vi "Configure_Voltage.vi"(6 "Measurement Type":T2(ring), 8 "error in (no error)":errorcluster, 9 "Resolution in Digits":T1(ring), 10 "Range":dbl=1.2, 11 "NI-DMM in":refnum<class "niDMM.lvclass">) -> (0 "error out":errorcluster, 3 "NI-DMM out":refnum<class "niDMM.lvclass">)   [LabVIEW 2021, in "niDMM.lvclass"]
uses:
  niDMM.lvclass
  niDMM.lvclass/niDMM.ctl
  <instrlib>/niDMM/nidmm.llb/niDMM Resolution in Digits.ctl
  <instrlib>/niDMM/nidmm.llb/niDMM Configure Measurement Digits.vi
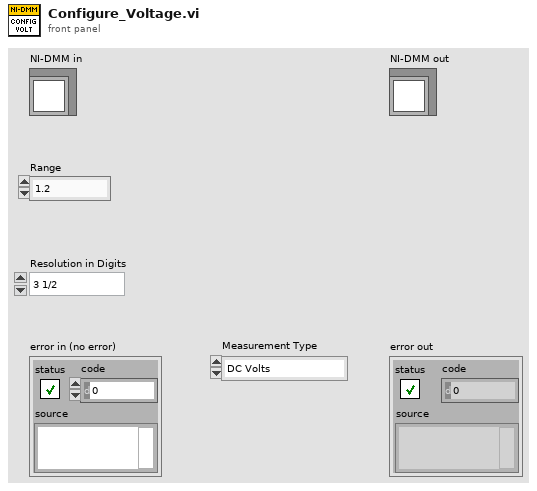
[diagram p1: front panel]
types:
  T1 = enum32{"3 1/2", "4 1/2", "5 1/2", "6 1/2", "7 1/2"}
  T2 = enum32{"DC Volts", "AC Volts", "DC Current", "AC Current", "2-wire Resistance", "4-wire Resistance", "Diode", "Frequency", "Period", "AC Volts DC Coupled", "Capacitance", "Inductance", "Temperature"}
  T3 = typedef "niDMM Resolution in Digits.ctl" = dbl
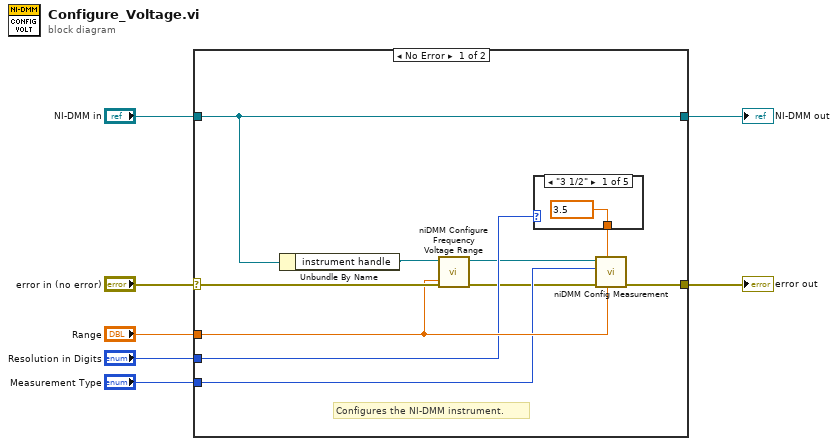
[diagram p0: block diagram]
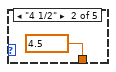
[diagram p2: hidden frame]
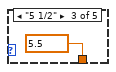
[diagram p3: hidden frame]
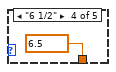
[diagram p4: hidden frame]
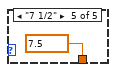
[diagram p5: hidden frame]
diagram:
  n1 = case shown="No Error" "error in (no error)" {
    selector: "error in (no error)" -> [w17 w23]
    tunnel: [w16 w23] -> w6
    tunnel: "NI-DMM in" -> [w12 w24]
    tunnel: [w12 w24] -> w4
    tunnel: "Range" -> [w15 _]
    tunnel: "Resolution in Digits" -> [w14 _]
    tunnel: "Measurement Type" -> [w13 _]
    frame No Error {
      # "Configures the NI-DMM instrument."
      n2 = Unbundle By Name(w12) -> ("instrument handle"=w11:refnum<k15>)
      n3 = call <instrlib>:"niDMM Configure Frequency Voltage Range.vi"("Frequency Voltage Range"=w15, "error in (no error)"=w17, "instrument handle"=w11) -> ("error out"=w8:errorcluster, "instrument handle out"=w9:refnum<k15>)  [unwired: 7 in]
      n4 = case shown="\"3 1/2\"" w14 {
        tunnel: [w18 w19 w20 w21 w22] -> w10
        frame "3 1/2" {
          w18 = T3 3.5 items=["3 1/2"=3.5, "4 1/2"=4.5, "5 1/2"=5.5, "6 1/2"=6.5, "7 1/2"=7.5] ("Resolution in Digits")
        }
        frame "4 1/2" {
          w19 = T3 4.5 items=["3 1/2"=3.5, "4 1/2"=4.5, "5 1/2"=5.5, "6 1/2"=6.5, "7 1/2"=7.5] ("Resolution in Digits")
        }
        frame "5 1/2" {
          w20 = T3 5.5 items=["3 1/2"=3.5, "4 1/2"=4.5, "5 1/2"=5.5, "6 1/2"=6.5, "7 1/2"=7.5] ("Resolution in Digits")
        }
        frame "6 1/2" {
          w21 = T3 6.5 items=["3 1/2"=3.5, "4 1/2"=4.5, "5 1/2"=5.5, "6 1/2"=6.5, "7 1/2"=7.5] ("Resolution in Digits")
        }
        frame "7 1/2" {
          w22 = T3 7.5 items=["3 1/2"=3.5, "4 1/2"=4.5, "5 1/2"=5.5, "6 1/2"=6.5, "7 1/2"=7.5] ("Resolution in Digits")
        }
      }
      n5 = call-poly <instrlib>:"niDMM Config Measurement.vi"("Range"=w15, "Resolution in Digits"=w10, "error in (no error)"=w8, "Function"=w13, "instrument handle"=w9) -> ("error out"=w16:errorcluster)  [unwired: 5 in, 1 out]
    }
    frame Error {
    }
  }
  "error out" <- w6
  "NI-DMM out" <- w4
